vi "tsa_AR Predictor (B).vi"(0 "Response signal":dbl[](array[numeric]) format="%.2f", 1 "not R matrix":bool, 3 "order":i32=4, 4 "block size":i32=1000) -> (5 "Backward Matrix":dbl[][](array[numeric]) format="%.2f", 6 "Backward Vector":dbl[](array[numeric]) format="%.2f")   [LabVIEW 2020, in "NI_AALPro.lvlib"]
uses:
  NI_AALPro.lvlib
  Real A x B.vi
  A x Vector.vi
  NI_AALBase.lvlib
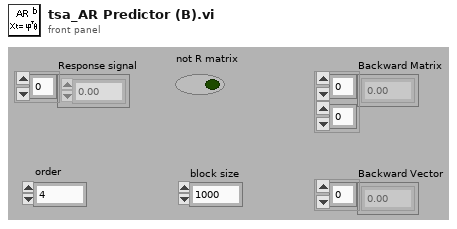
[diagram p1: front panel]
types:
  T1 = typedef "NI_Matrix.lvlib/RealMatrix.ctl" = dbl[][]
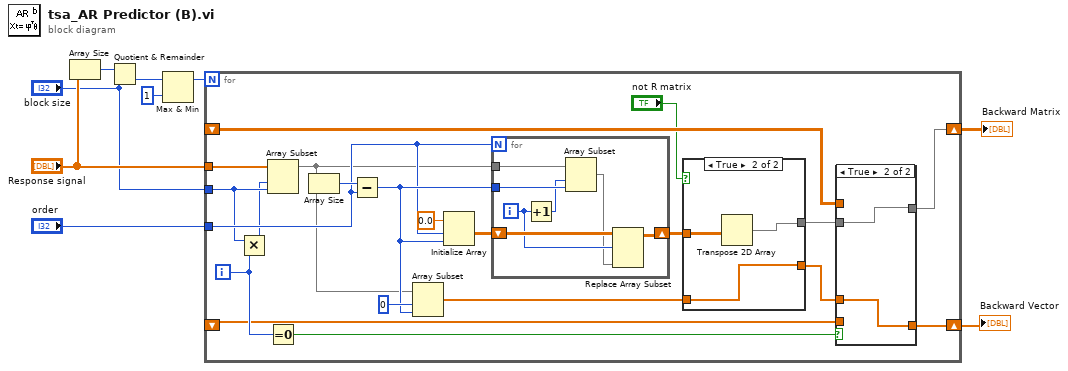
[diagram p0: block diagram]
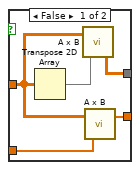
[diagram p2: hidden frame]
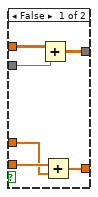
[diagram p3: hidden frame]
diagram:
  n1 = Array Size(array="Response signal") -> (size(s)=w8:i32)
  n2 = Quotient & Remainder(x=w8, y="block size") -> (floor(x/y)=w7:i32)  [unwired: 1 out]
  n3 = Max & Min(x=w7, y=1) -> (max(x,y)=w5:i32)  [unwired: 1 out]
  n4 = for {
    N: w5 -> [_]
    tunnel: "Response signal" -> [w24]
    tunnel: "order" -> [w25]
    tunnel: "block size" -> [w22]
    shift-right: [w16] -> w1
    shift-left: _ -> [w17]
    shift-right: [w14] -> w2
    shift-left: _ -> [w12]
    i -> [w20]
    n5 = Multiply(x=w22, y=w20) -> (x*y=w21:i32)
    n6 = Array Subset(array=w24, index=w21, length=w22) -> (w23:dbl[])
    n7 = Equal To 0?(x=w20) -> (x = 0?=w19:bool)
    n8 = Array Size(array=w23) -> (size(s)=w30:i32)
    n9 = Subtract(x=w30, y=w25) -> (x-y=w26:i32)
    n10 = Array Subset(array=w23, index=0, length=w26) -> (w15:dbl[])
    n11 = Initialize Array(0.0 ("element"), w25, w26) -> (w27:dbl[][])
    n12 = for {
      N: w25 -> [_]
      tunnel: w23 -> [w53]
      tunnel: w26 -> [w52]
      shift-right: [w49] -> w11
      shift-left: w27 -> [w50]
      i -> [w48]
      n13 = Increment(x=w48) -> (x+1=w51:i32)
      n14 = Array Subset(array=w53, index=w51, length=w52) -> (w47:dbl[])
      n15 = Replace Array Subset(array=w50, new element=w47, index (row)=w48) -> (w49:dbl[][])  [unwired: 1 in]
    }
    n16 = case shown="True" "not R matrix" {
      tunnel: [w35 w36] -> w18
      tunnel: w15 -> [w33 w38]
      tunnel: [w32 w38] -> w13
      tunnel: w11 -> [w31 w37]
      frame False {
        n17 = Transpose 2D Array(2D array=w31) -> (transposed array=w34:dbl[][])
        n18 = call-poly "A x B.vi"("B"=w34, "A"=w31) -> ("A x B"=w35:T1)  [unwired: 1 out]
        n19 = call-poly "A x B.vi"("Vector"=w33, "A"=w31) -> ("A x Vector"=w32:dbl[])  [unwired: 1 out]
      }
      frame True {
        n20 = Transpose 2D Array(2D array=w37) -> (transposed array=w36:dbl[][])
      }
    }
    n21 = case shown="True" w19 {
      tunnel: w17 -> [w44 _]
      tunnel: [w43 w46] -> w16
      tunnel: w18 -> [w42 w46]
      tunnel: w12 -> [w41 _]
      tunnel: [w40 w45] -> w14
      tunnel: w13 -> [w39 w45]
      frame False {
        n22 = Add(x=w44, y=w42) -> (x+y=w43:dbl[][])
        n23 = Add(x=w41, y=w39) -> (x+y=w40:dbl[])
      }
      frame True {
      }
    }
  }
  "Backward Matrix" <- w1
  "Backward Vector" <- w2
